vi "EdmundsFilterWheel.vi"() -> ()   [LabVIEW 2018]
uses:
  C:/Users/aspitarl/Git/MHDLab/Acquisition/Instruments/Edmunds Filter Wheel/OptecHID_FilterWheelAPI.dll
  OptecHID_FilterWheelAPI.dll
panel:
  out "Set Filter Name":string="775     "
  out "Current Filter Name":string
  out "Filter Names":string[](array[string])
  in  "Send":bool
  in  "Set Position":u32=1 min=1 max=5 step=1
  in  "stop":bool
  out "CurrentPosition":i16
  out "# Filter Wheels":i32
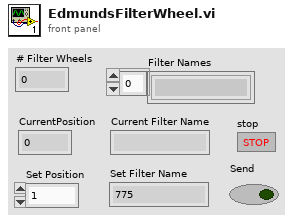
[diagram p1: front panel]
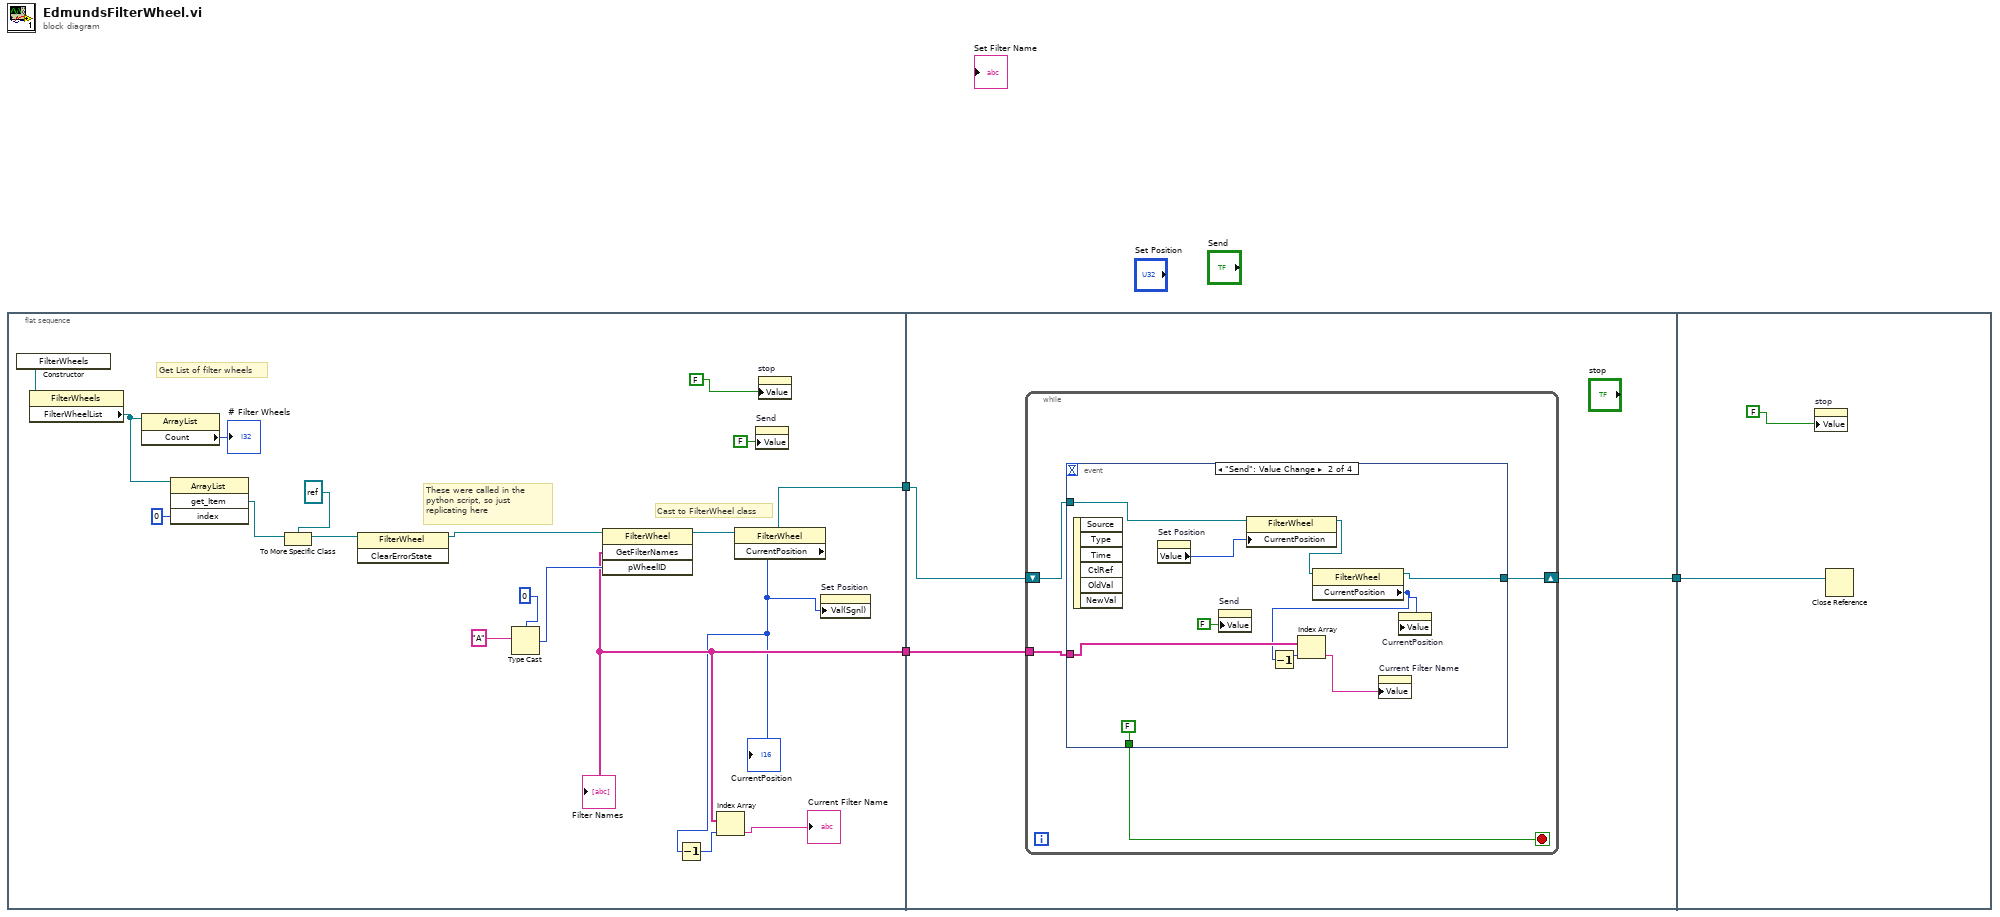
[diagram p0: block diagram]
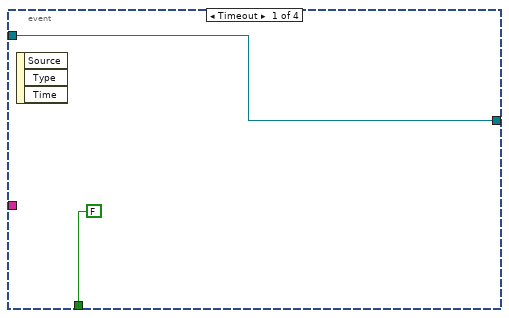
[diagram p2: hidden frame]
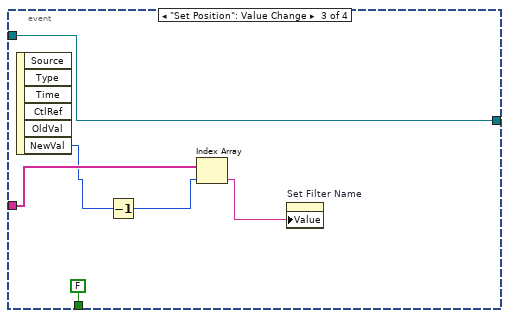
[diagram p3: hidden frame]
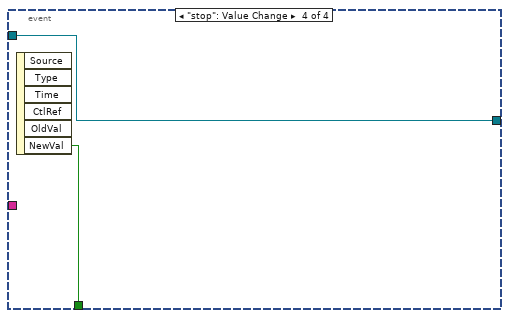
[diagram p4: hidden frame]
diagram:
  n1 = flat-sequence {
    tunnel: [w16] -> w3
    tunnel: [w6] -> w1
    tunnel: w3 -> [w25]
    tunnel: [w24] -> w2
    tunnel: w1 -> [w23]
    tunnel: w2 -> [w51]
    frame #0 {
      # "These were called in the python script, so just replicating here"
      # "Cast to FilterWheel class"
      # "Get List of filter wheels"
      n2 = constructor class="FilterWheels"() -> (reference out=w22:refnum<k24>)  [unwired: 3 in, 2 out]
      n3 = property class="FilterWheels"(reference=w22) -> ("FilterWheelList"=w20:refnum<k24>)  [unwired: 1 in, 2 out]
      n4 = property class="ArrayList"(reference=w20) -> ("Count"=→"# Filter Wheels":i32)  [unwired: 1 in, 2 out]
      n5 = invoke class="ArrayList" method="get_Item"(reference=w20, "index"=0) -> ("get_Item"=w18:refnum<k24>)  [unwired: 2 in, 3 out]
      n6 = To More Specific Class(target class=refnum<k24> refnum ("reference out"), reference=w18) -> (specific class reference=w15:refnum<k24>)  [unwired: 1 in, 1 out]
      n7 = invoke class="FilterWheel" method="ClearErrorState"(reference=w15) -> (reference out=w14:refnum<k24>)  [unwired: 2 in, 2 out]
      n8 = Type Cast(type=u8 0, x="A") -> (*(type *) &x=w9:u8)
      n9 = invoke class="FilterWheel" method="GetFilterNames"(reference=w14, "pWheelID"=w9) -> (reference out=w13:refnum<k24>, "GetFilterNames"=w6:string[])  [unwired: 2 in, 2 out]
      "Filter Names" <- w6
      n10 = property class="FilterWheel"(reference=w13) -> (reference out=w16:refnum<k24>, "CurrentPosition"=w5:i16)  [unwired: 1 in, 1 out]
      "CurrentPosition" <- w5
      n11 = Decrement(x=w5) -> (x-1=w4:i16)
      n12 = Index Array(array=w6, index=w4) -> (element=→"Current Filter Name":string)
      n13 = property on="Send" class="Bool (strict)"("Value"=FALSE ("Send")) -> ()  [unwired: 2 in, 2 out]
      n14 = property on="stop" class="Bool (strict)"("Value"=FALSE) -> ()  [unwired: 2 in, 2 out]
      n15 = property on="Set Position" class="DigNum (strict)"("Val(Sgnl)"=w5) -> ()  [unwired: 2 in, 2 out]
    }
    frame #1 {
      n16 = while {
        shift-right: [w27] -> w24
        shift-left: w25 -> [w28]
        tunnel: w23 -> [w26]
        stop <- w29 stop-if-true
        n17 = event shown="[1] \"Send\": Value Change" {
          selector: _ -> [_ _ _ _]
          dyn-events: _ -> [_ _ _ _]
          timeout: _ -> [_ _ _ _]
          tunnel: [FALSE ("NewVal") FALSE ("NewVal") FALSE ("NewVal") w49] -> w29
          tunnel: w28 -> [w30 w39 w45 w48]
          tunnel: [w30 w37 w45 w48] -> w27
          tunnel: w26 -> [_ w35 w46 _]
          event Timeout {
            n18 = event-data() -> ()  [unwired: 1 in, 3 out]
          }
          event "Send": Value Change {
            n19 = event-data() -> ()  [unwired: 1 in, 6 out]
            n20 = property on="Set Position" class="DigNum (strict)"() -> ("Value"=w40:u32)  [unwired: 2 in, 2 out]
            n21 = property on="Send" class="Bool (strict)"("Value"=FALSE ("Send")) -> ()  [unwired: 2 in, 2 out]
            n22 = property class="FilterWheel"(reference=w39, "CurrentPosition"=w40) -> (reference out=w38:refnum<k24>)  [unwired: 1 in, 1 out]
            n23 = property class="FilterWheel"(reference=w38) -> (reference out=w37:refnum<k24>, "CurrentPosition"=w33:i16)  [unwired: 1 in, 1 out]
            n24 = Decrement(x=w33) -> (x-1=w32:i16)
            n25 = Index Array(array=w35, index=w32) -> (element=w34:string)
            n26 = property on="Current Filter Name" class="Str"("Value"=w34) -> ()  [unwired: 2 in, 2 out]
            n27 = property on="CurrentPosition" class="DigNum (strict)"("Value"=w33) -> ()  [unwired: 2 in, 2 out]
          }
          event "Set Position": Value Change {
            n28 = event-data() -> ("NewVal"=w43:u32)  [unwired: 1 in, 5 out]
            n29 = Decrement(x=w43) -> (x-1=w42:u32)
            n30 = Index Array(array=w46, index=w42) -> (element=w47:string)
            n31 = property on="Set Filter Name" class="Str"("Value"=w47) -> ()  [unwired: 2 in, 2 out]
          }
          event "stop": Value Change {
            n32 = event-data() -> ("NewVal"=w49:bool)  [unwired: 1 in, 5 out]
          }
        }
      }
    }
    frame #2 {
      n33 = property on="stop" class="Bool (strict)"("Value"=FALSE) -> ()  [unwired: 2 in, 2 out]
      n34 = Close Reference(reference=w51) -> ()  [unwired: 1 in, 1 out]
    }
  }
